vi "RedP_api -- V1.vi"(5 "red pita ip Address":string="146.201.232.88", 6 "delay-circle(msec)":i64, 7 "MFLI frontend action":T2, 8 "Error In":errorcluster, 10 "Freq IN (Hz)":dbl=40000.0 format="%#_13g", 11 "RedPitaSettings":T1) -> (0 "Error Out":errorcluster, 1 "z out (V)":cdb, 2 "Freq out (Hz)":dbl=40000.0 format="%#_13g", 3 "RedPitaSettings OUT":T1)   [LabVIEW 2018]
uses:
  MFLI frontend action.ctl
  RedPitaSettings.ctl
  NHMFL_Core/Libraries/Red Pitaya/RP Core/RP Transceiver/RP Transceiver.lvclass
  Users/arkady/Desktop/ado/github/NHMFL_Core/Libraries/Red Pitaya/RP Core/RP Instrument/RP Instrument.lvclass
  NHMFL_Core/Libraries/Red Pitaya/RP Core/RP Transceiver/Receiver format.ctl
  NHMFL_Core/Libraries/Red Pitaya/RP Core/RP Instrument/RP Instrument.lvclass/RP Instrument.ctl
  NHMFL_Core/Libraries/Red Pitaya/RP Core/RP Transceiver/RP Transceiver.lvclass/RP Transceiver.ctl
  NHMFL_Core/Libraries/Red Pitaya/RP Core/RP Instrument/Write Status check delay.vi
  NHMFL_Core/Libraries/Red Pitaya/RP Core/RP Transceiver/Write Receiver format.vi
  NHMFL_Core/Libraries/Red Pitaya/RP Core/RP Instrument/Write DDS delay.vi
  NHMFL_Core/Libraries/Red Pitaya/RP Core/RP Instrument/Write Server address.vi
panel:
  in  "timeconstant (s)":dbl=0.006
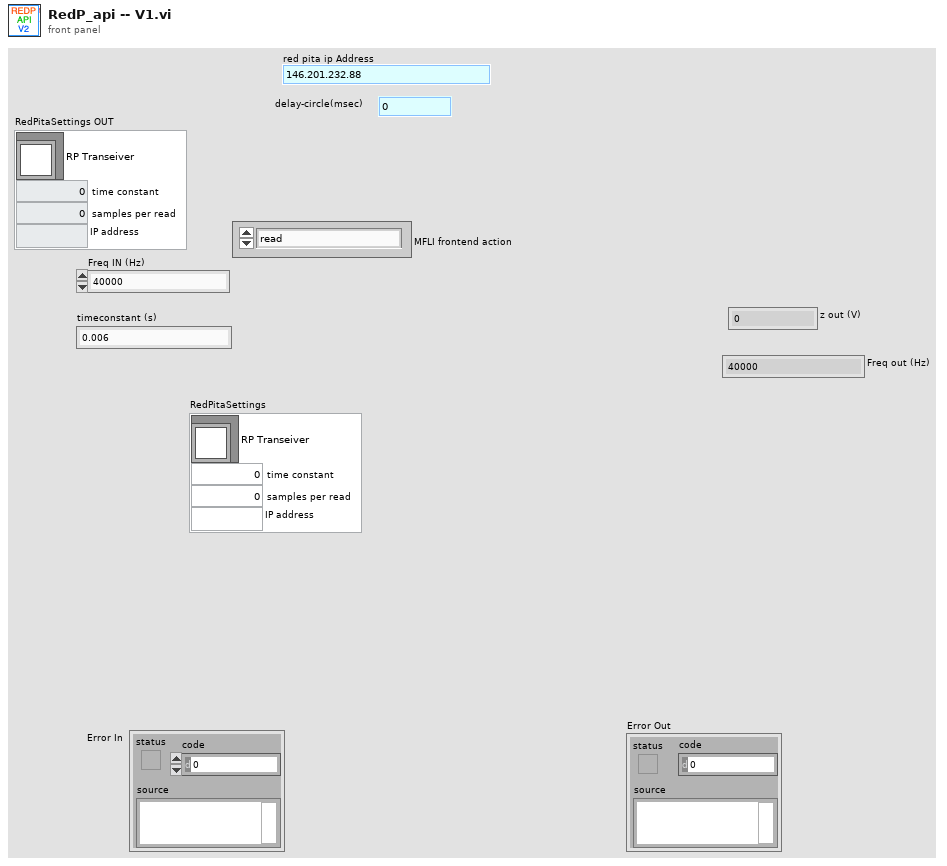
[diagram p1: front panel]
types:
  T1 = typedef "RedPitaSettings.ctl" = cluster{"time constant":dbl, "RP Transeiver":refnum<class "RP Transceiver.lvclass">, "samples per read":i32, "IP address":string}
  T2 = typedef "MFLI frontend action.ctl" = enum16{"read", "writeread", "open", "close", "write"}
  T3 = typedef "Receiver format.ctl" = enum16{"X-Y-F", "F-X-Y", "X-Y", "X"}
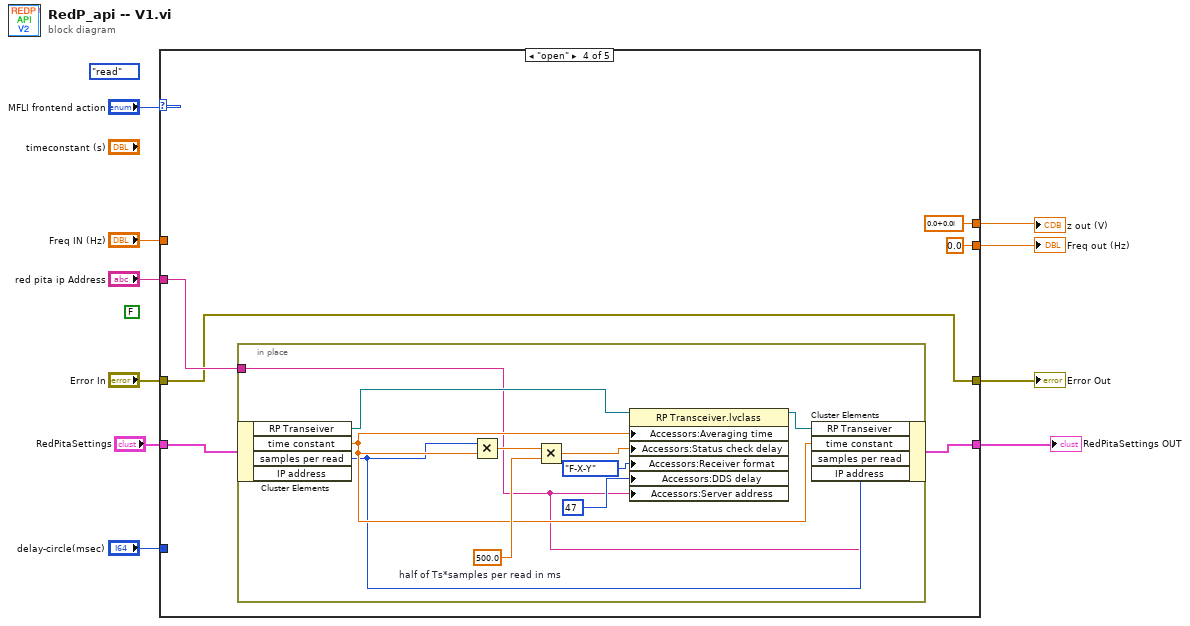
[diagram p0: block diagram]
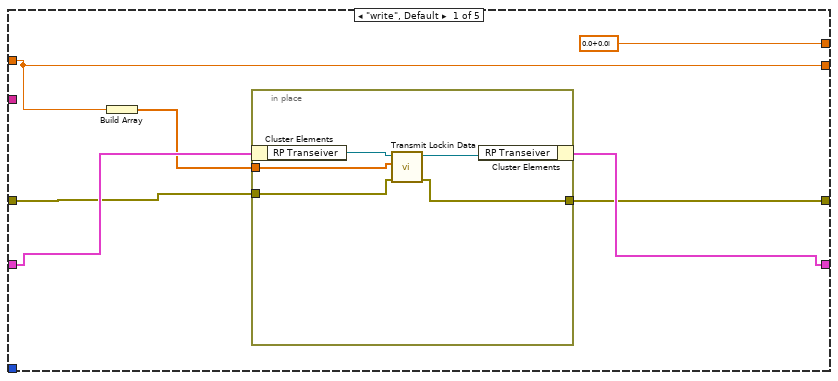
[diagram p2: hidden frame]
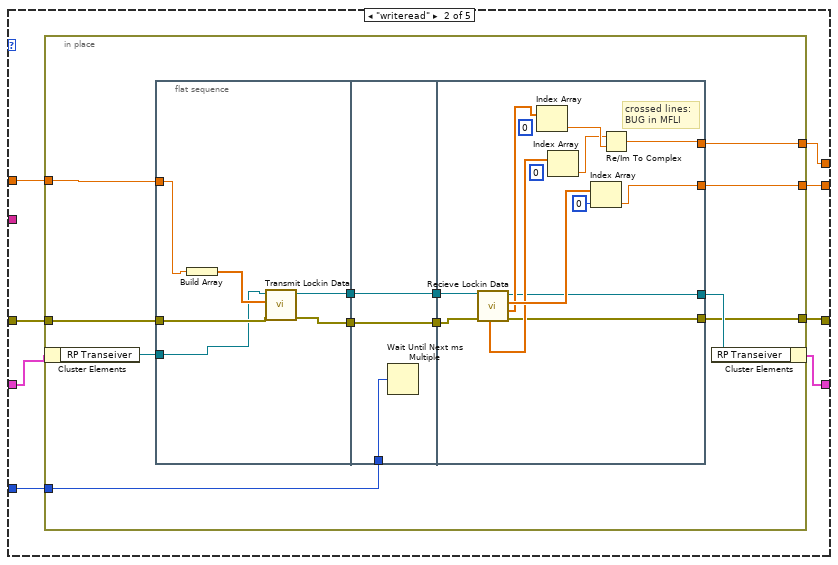
[diagram p3: hidden frame]
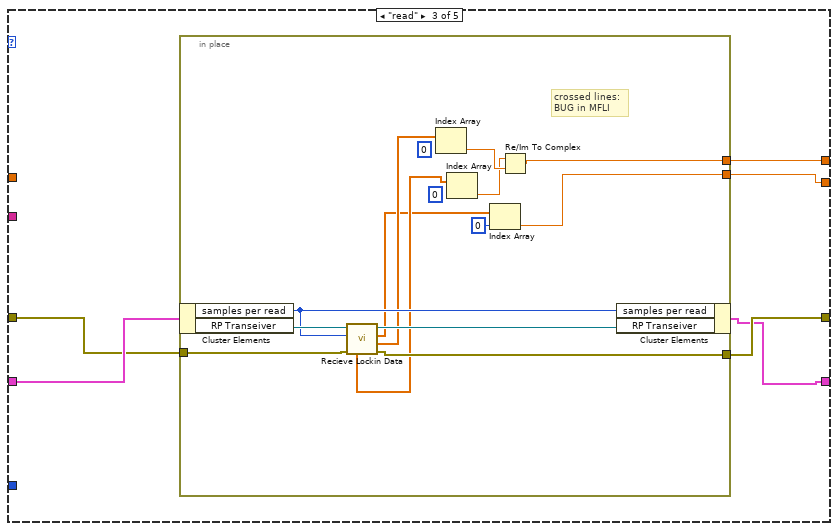
[diagram p4: hidden frame]
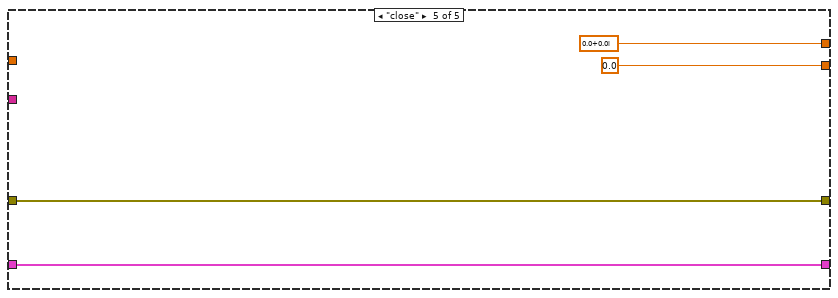
[diagram p5: hidden frame]
diagram:
  (unwired) MFLI_frontend_action."read" ("MFLI frontend action")
  (unwired) FALSE
  n1 = case shown="\"open\"" "MFLI frontend action" {
    tunnel: [w13 w23 w66 w83 w100] -> w10
    tunnel: [cdb 0.0+0.0i w26 w69 cdb 0.0+0.0i cdb 0.0+0.0i] -> w9
    tunnel: "Error In" -> [w14 w30 w67 w83 w100]
    tunnel: [w11 w27 w64 0.0 ("Freq (Hz)") 0.0 ("Freq (Hz)")] -> w7
    tunnel: "red pita ip Address" -> [_ _ _ w85 _]
    tunnel: "Freq IN (Hz)" -> [w11 w29 _ _ _]
    tunnel: "delay-circle(msec)" -> [_ w28 _ _ _]
    tunnel: "RedPitaSettings" -> [w16 w25 w68 w86 w99]
    tunnel: [w15 w24 w65 w84 w99] -> w1
    frame "write", Default {
      n2 = Build Array(w11) -> (w12:dbl[])
      n3 = in-place {
        in-place-border: w14 -> [w20]
        in-place-border: [w19] -> w13
        in-place-border: w12 -> [w18]
        n4 = in-place-cluster #1(w16) -> ("RP Transeiver"=w22:refnum<class "RP Transceiver.lvclass">)
        n5 = call-dynamic "Transmit Lockin Data.vi"("error in (no error)"=w20, "Data"=w18, "RP Transceiver in"=w22) -> ("error out"=w19:errorcluster, "RP Transceiver out"=w21:refnum<class "RP Transceiver.lvclass">)  [unwired: 6 in, 1 out]
        n6 = in-place-cluster #1("RP Transeiver"=w21) -> (w15:T1)
      }
    }
    frame "writeread" {
      n7 = in-place {
        in-place-border: w30 -> [w38]
        in-place-border: w29 -> [w37]
        in-place-border: w28 -> [w36]
        in-place-border: [w35] -> w27
        in-place-border: [w34] -> w26
        in-place-border: [w31] -> w23
        n8 = in-place-cluster #2(w25) -> ("RP Transeiver"=w33:refnum<class "RP Transceiver.lvclass">)
        n9 = flat-sequence {
          tunnel: w38 -> [w46]
          tunnel: w37 -> [w48]
          tunnel: [w45] -> w42
          tunnel: [w44] -> w41
          tunnel: w33 -> [w43]
          tunnel: w42 -> [w51]
          tunnel: [w51] -> w40
          tunnel: w36 -> [w50]
          tunnel: [w49] -> w39
          tunnel: w41 -> [w49]
          tunnel: w40 -> [w53]
          tunnel: [w59] -> w35
          tunnel: [w63] -> w34
          tunnel: w39 -> [w62]
          tunnel: [w54] -> w32
          tunnel: [w52] -> w31
          frame #0 {
            n10 = Build Array(w48) -> (w47:dbl[])
            n11 = call-dynamic "Transmit Lockin Data.vi"("error in (no error)"=w46, "Data"=w47, "RP Transceiver in"=w43) -> ("error out"=w45:errorcluster, "RP Transceiver out"=w44:refnum<class "RP Transceiver.lvclass">)  [unwired: 6 in, 1 out]
          }
          frame #1 {
            n12 = Wait Until Next ms Multiple(millisecond multiple=w50) -> ()  [unwired: 1 out]
          }
          frame #2 {
            (unwired) 0 ("index")
            (unwired) 0 ("index")
            # "crossed lines:\nBUG in MFLI"
            n13 = call-dynamic "Recieve Lockin Data.vi"("error in (no error)"=w53, "RP Lockin in"=w62) -> ("error out"=w52:errorcluster, "Volatge X out"=w58:dbl[], "Frequency out"=w61:dbl[], "RP Lockin out"=w54:refnum<class "RP Transceiver.lvclass">, "Volatge Y out"=w56:dbl[])  [unwired: 3 in, 2 out]
            n14 = Index Array(array=w58) -> (element=w57:dbl)  [unwired: 1 in]
            n15 = Index Array(array=w56) -> (element=w55:dbl)  [unwired: 1 in]
            n16 = Index Array(array=w61, index=0) -> (element=w59:dbl)
            n17 = Re/Im To Complex(1:w57, 2:w55) -> (0:w63:cdb)
          }
        }
        n18 = in-place-cluster #2("RP Transeiver"=w32) -> (w24:T1)
      }
    }
    frame "read" {
      n19 = in-place {
        in-place-border: [w71] -> w69
        in-place-border: w67 -> [w81]
        in-place-border: [w80] -> w66
        in-place-border: [w70] -> w64
        (unwired) 0 ("index")
        (unwired) 0 ("index")
        # "crossed lines:\nBUG in MFLI"
        n20 = in-place-cluster #3(w68) -> ("samples per read"=w78:i32, "RP Transeiver"=w82:refnum<class "RP Transceiver.lvclass">)
        n21 = call-dynamic "Recieve Lockin Data.vi"("error in (no error)"=w81, "Points to read"=w78, "RP Lockin in"=w82) -> ("error out"=w80:errorcluster, "Volatge X out"=w76:dbl[], "Frequency out"=w72:dbl[], "RP Lockin out"=w79:refnum<class "RP Transceiver.lvclass">, "Volatge Y out"=w75:dbl[])  [unwired: 2 in, 2 out]
        n22 = Index Array(array=w76) -> (element=w74:dbl)  [unwired: 1 in]
        n23 = Index Array(array=w75) -> (element=w73:dbl)  [unwired: 1 in]
        n24 = Index Array(array=w72, index=0) -> (element=w70:dbl)
        n25 = Re/Im To Complex(1:w74, 2:w73) -> (0:w71:cdb)
        n26 = in-place-cluster #3("samples per read"=w78, "RP Transeiver"=w79) -> (w65:T1)
      }
    }
    frame "open" {
      n27 = in-place {
        in-place-border: w85 -> [w89]
        w97 = 500.0  # half of Ts*samples per read in ms
        n28 = in-place-cluster #4(w86) -> ("RP Transeiver"=w93:refnum<class "RP Transceiver.lvclass">, "time constant"=w91:dbl, "samples per read"=w90:i32)  [unwired: 1 out]
        n29 = Multiply(x=w90, y=w91) -> (x*y=w98:dbl)
        n30 = Multiply(x=w98, y=w97) -> (x*y=w96:dbl)
        n31 = property class="RP Transceiver.lvclass"(reference=w93, "Accessors:Averaging time"=w91, "Accessors:Status check delay"=w96, "Accessors:Receiver format"=Receiver_format."F-X-Y" ("Receiver format"), "Accessors:DDS delay"=u32 47 ("DDS delay"), "Accessors:Server address"=w89) -> (reference out=w92:refnum<class "RP Transceiver.lvclass">)  [unwired: 1 in, 1 out]
        n32 = in-place-cluster #4("RP Transeiver"=w92, "time constant"=w91, "samples per read"=w90, "IP address"=w89) -> (w84:T1)
      }
    }
    frame "close" {
    }
  }
  "Error Out" <- w10
  "z out (V)" <- w9
  "Freq out (Hz)" <- w7
  "RedPitaSettings OUT" <- w1
